vi "QUBE2 RW.vi"(0 "QFLEX Cluster In":T1={"Error"={"status"=FALSE, "code"=0, "source"=""}, "CS DO Ref"={"myRIO Reference"={"myRIO Model"=enum."Unknown", "myRIO Hardware Reference"={"Generic FPGA Reference"=refnum, "Allow multiple opens"=FALSE}}, "DIO Channels List"=[]}, "SPI Ref"={"myRIO Reference"={"myRIO Model"=enum."Unknown", "myRIO Hardware Reference"={"Generic FPGA Reference"=refnum, "Allow multiple opens"=FALSE}}, "SPI Channels Enum"=enum."Not Connected", "SPI Configuration"={"Frequency [Hz]"=0.0, "Clock Phase"=enum."Leading", "Clock Polarity"=enum."Low", "Data Direction"=enum."Most significant bit first", "Frame Length"=8}}} {"SPI Ref"."SPI Configuration"."Frame Length" min=1 max=16}, 5 "LED Color":u32(colorbox)=16711680, 9 "Motor Voltage":dbl, 11 "Reset":bool) -> (3 "Hardware Info":u16[](array[numeric]), 4 "QFLEX Cluster Out":T1={"Error"={"status"=FALSE, "code"=0, "source"=""}, "CS DO Ref"={"myRIO Reference"={"myRIO Model"=enum."Unknown", "myRIO Hardware Reference"={"Generic FPGA Reference"=refnum, "Allow multiple opens"=FALSE}}, "DIO Channels List"=[]}, "SPI Ref"={"myRIO Reference"={"myRIO Model"=enum."Unknown", "myRIO Hardware Reference"={"Generic FPGA Reference"=refnum, "Allow multiple opens"=FALSE}}, "SPI Channels Enum"=enum."Not Connected", "SPI Configuration"={"Frequency [Hz]"=0.0, "Clock Phase"=enum."Leading", "Clock Polarity"=enum."Low", "Data Direction"=enum."Most significant bit first", "Frame Length"=8}}} {"SPI Ref"."SPI Configuration"."Frame Length" min=1 max=16}, 6 "Encoder (counts)":i32[](array[numeric]), 8 "Encoders (rads)":dbl[](array[numeric]), 10 "Tachometer (rads/s)":dbl, 12 "Stall Error":bool, 15 "Motor Current (mA)":dbl)   [LabVIEW 2016]
uses:
  QFLEX myRIO.ctl
  <vilib>/myRIO/Instrument Drivers/Onboard IO/DIO/typedefs/DIO Reference.ctl
  <vilib>/myRIO/Common/Instrument Driver Framework/Utilities/typedefs/myRIO Generic Hardware Reference.ctl
  <vilib>/myRIO/Common/Instrument Driver Framework/Utilities/typedefs/Hardware Version Enum.ctl
  <vilib>/myRIO/Common/Instrument Driver Framework/Utilities/typedefs/myRIO v1.0 Reference.ctl
  <vilib>/myRIO/Common/Instrument Driver Framework/Utilities/typedefs/Generic FPGA Reference.ctl
  <vilib>/myRIO/Common/Instrument Driver Framework/myRIO v1.0/DIO/typedefs/DIO Channels List.ctl
  <vilib>/myRIO/Common/Instrument Driver Framework/myRIO v1.0/DIO/typedefs/DIO Channels Enum.ctl
  <vilib>/myRIO/Instrument Drivers/Onboard IO/SPI/typedefs/SPI Reference.ctl
  <vilib>/myRIO/Common/Instrument Driver Framework/myRIO v1.0/SPI/typedefs/SPI Channels Enum.ctl
  <vilib>/myRIO/Instrument Drivers/Onboard IO/SPI/typedefs/SPI Configuration.ctl
  <vilib>/myRIO/Common/Instrument Driver Framework/myRIO v1.0/SPI/typedefs/SPI Clock Phase.ctl
  <vilib>/myRIO/Common/Instrument Driver Framework/myRIO v1.0/SPI/typedefs/SPI Clock Polarity.ctl
  <vilib>/myRIO/Common/Instrument Driver Framework/myRIO v1.0/SPI/typedefs/SPI Data Direction.ctl
  <vilib>/myRIO/Common/Instrument Driver Framework/myRIO v1.0/SPI/typedefs/SPI Frame Length.ctl
  <vilib>/Utility/error.llb/Error Cluster From Error Code.vi
  <vilib>/myRIO/Common/Instrument Driver Framework/myRIO v1.0/DIO/vis/myRIO v1.0 Write DIO.vi
  <vilib>/myRIO/Common/Instrument Driver Framework/myRIO v1.0/SPI/vis/myRIO v1.0 Write Read SPI.vi
  <vilib>/myRIO/Instrument Drivers/Onboard IO/SPI/SPI.lvlib
  <vilib>/myRIO/Instrument Drivers/Onboard IO/DIO/DIO.lvlib
panel:
  out "Stall Detect":bool
  out "Amp Error":bool
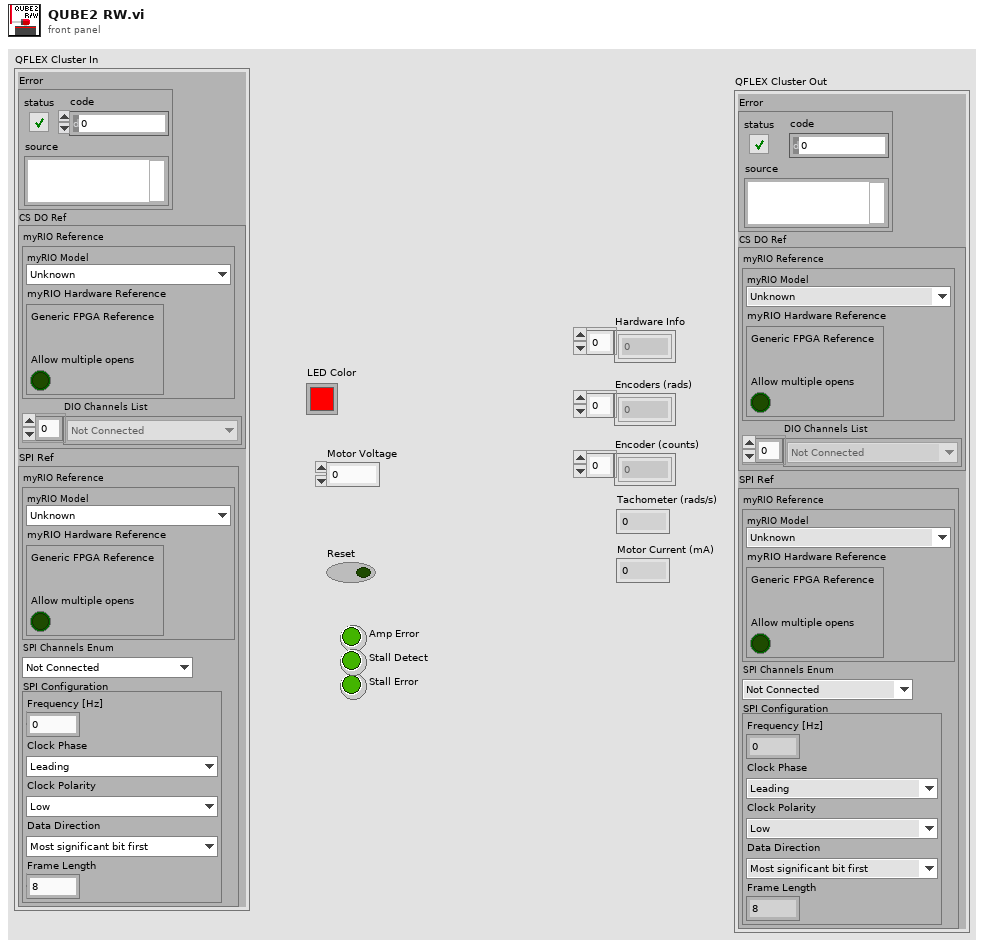
[diagram p1: front panel]
types:
  T1 = typedef "QFLEX myRIO.ctl" = cluster{"Error":errorcluster, "CS DO Ref":T2, "SPI Ref":T9}
  T2 = typedef "DIO.lvlib/DIO Reference.ctl" = cluster{"myRIO Reference":T3, "DIO Channels List":T7}
  T3 = typedef "myRIO Generic Hardware Reference.ctl" = cluster{"myRIO Model":T4, "myRIO Hardware Reference":T5}
  T4 = typedef "Hardware Version Enum.ctl" = enum16{"Unknown", "myRIO-1900", "myRIO-1950", "roboRIO", "NI ELVIS RIO CM"}
  T5 = typedef "myRIO v1.0 Reference.ctl" = cluster{"Generic FPGA Reference":T6, "Allow multiple opens":bool}
  T6 = typedef "Generic FPGA Reference.ctl" = refnum<k20>
  T7 = typedef "DIO Channels List.ctl" = T8[]
  T8 = typedef "DIO Channels Enum.ctl" = enum16{"Not Connected", "C/DIO0", "C/DIO1", "C/DIO2", "C/DIO3", "C/DIO4", "C/DIO5", "C/DIO6", "C/DIO7", "A/DIO0", "A/DIO1", "A/DIO2", "A/DIO3", "A/DIO4", "A/DIO5", "A/DIO6", "A/DIO7", "A/DIO8", "A/DIO9", "A/DIO10", "A/DIO11", "A/DIO12", "A/DIO13", "A/DIO14", "A/DIO15", "B/DIO0", "B/DIO1", "B/DIO2", "B/DIO3", "B/DIO4", "B/DIO5", "B/DIO6", "B/DIO7", "B/DIO8", "B/DIO9", "B/DIO10", "B/DIO11", "B/DIO12", "B/DIO13", "B/DIO14", "B/DIO15", "LED0", "LED1", "LED2", "LED3", "Button0", "DIO/DIO0", "DIO/DIO1", "DIO/DIO2", "DIO/DIO3", "DIO/DIO4", "DIO/DIO5", "DIO/DIO6", "DIO/DIO7", "DIO/DIO8", "DIO/DIO9", "SPI/CS0", "SPI/CS1", "SPI/CS2", "SPI/CS3", "LED RADIO (Green)", "LED RADIO (Red)", "LED COMM (Green)", "LED COMM (Red)", "LED MODE (Green)", "LED MODE (Red)"}
  T9 = typedef "SPI.lvlib/SPI Reference.ctl" = cluster{"myRIO Reference":T3, "SPI Channels Enum":T10, "SPI Configuration":T11}
  T10 = typedef "SPI Channels Enum.ctl" = enum16{"Not Connected", "A/SPI", "B/SPI", "SPI/SPI"}
  T11 = typedef "SPI.lvlib/SPI Configuration.ctl" = cluster{"Frequency [Hz]":dbl, "Clock Phase":T12, "Clock Polarity":T13, "Data Direction":T14, "Frame Length":T15}
  T12 = typedef "SPI Clock Phase.ctl" = enum8{"Leading", "Trailing"}
  T13 = typedef "SPI Clock Polarity.ctl" = enum8{"Low", "High"}
  T14 = typedef "SPI Data Direction.ctl" = enum8{"Most significant bit first", "Least significant bit first"}
  T15 = typedef "SPI Frame Length.ctl" = u8
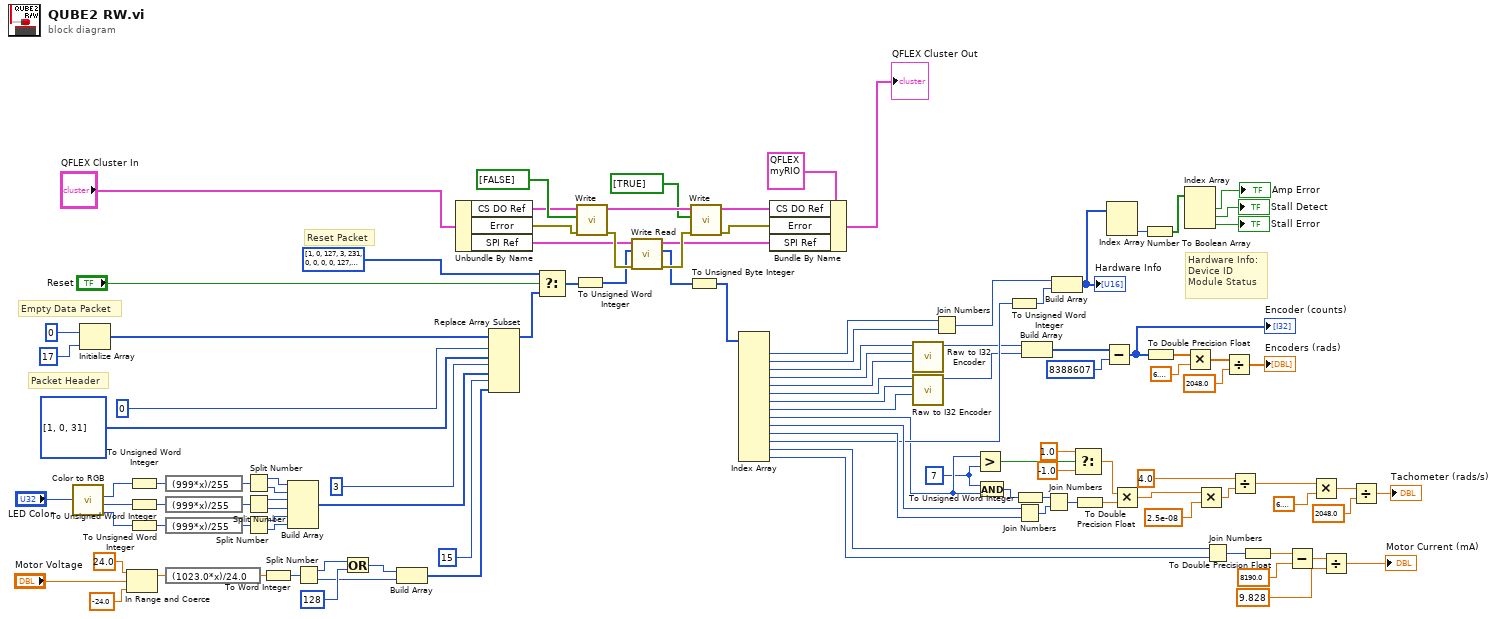
[diagram p0: block diagram]
diagram:
  w46 = u8 7 ("x")
  # "Reset Packet"
  # "Hardware Info:\nDevice ID\nModule Status"
  # "Empty Data Packet"
  # "Packet Header"
  n1 = call <vilib>:"Color to RGB.vi"("Color"="LED Color") -> ("R"=w107:u8, "G"=w100:u8, "B"=w99:u8)  [unwired: 1 out]
  n2 = Initialize Array(u8 0, 17 ("dimension size")) -> (w111:u8[])
  n3 = In Range and Coerce(upper limit=24.0, x="Motor Voltage", lower limit=-24.0) -> (coerced(x)=w36:dbl)  [unwired: 1 out]
  n4 = To Unsigned Word Integer(number=w107) -> (unsigned 16bit integer=w106:u16)
  n5 = To Unsigned Word Integer(number=w100) -> (unsigned 16bit integer=w104:u16)
  n6 = To Unsigned Word Integer(number=w99) -> (unsigned 16bit integer=w102:u16)
  n7 = expression code="(999*x)/255"(w106) -> (w105:u16)
  n8 = expression code="(999*x)/255"(w104) -> (w103:u16)
  n9 = expression code="(999*x)/255"(w102) -> (w101:u16)
  n10 = expression code="(1023.0*x)/24.0"(w36) -> (w89:dbl)
  n11 = Split Number(x=w105) -> (hi(x)=w93:u8, lo(x)=w94:u8)
  n12 = Split Number(x=w103) -> (hi(x)=w95:u8, lo(x)=w96:u8)
  n13 = Split Number(x=w101) -> (hi(x)=w97:u8, lo(x)=w98:u8)
  n14 = To Word Integer(number=w89) -> (16bit integer=w70:i16)
  n15 = Build Array(w93, w94, w95, w96, w97, w98) -> (w91:u8[])
  n16 = Split Number(x=w70) -> (hi(x)=w88:u8, lo(x)=w86:u8)
  n17 = Or(x=w88, y=u8 128) -> (x .or. y?=w85:u8)
  n18 = Build Array(w85, w86) -> (w69:u8[])
  n19 = Unbundle By Name("QFLEX Cluster In") -> ("CS DO Ref"=w23:T2, "Error"=w22:errorcluster, "SPI Ref"=w21:T9)
  n20 = Replace Array Subset(array=w111, new element #1=u8[] [1, 0, 31], index #1=0 ("dimension size"), new element #2=w91, index #2=3 ("dimension size"), new element #3=w69, index #3=15 ("dimension size")) -> (w77:u8[])
  n21 = Select(t=u8[] [1, 0, 127, 3, 231, 0, 0, 0, 0, 127, 255, 255, 127, 255, 255, 0, 0], s="Reset", f=w77) -> (s? t:f=w28:u8[])
  n22 = To Unsigned Word Integer(number=w28) -> (unsigned 16bit integer=w25:u16[])
  n23 = call <vilib>:"Write.vi"("error in (no error)"=w22, "Values"=bool[] [FALSE], "DIO Ref In"=w23) -> ("error out"=w33:errorcluster, "DIO Ref Out"=w32:T2)  [unwired: 6 in]
  n24 = call <vilib>:"Write Read.vi"("error in (no error)"=w33, "Frames to Write"=w25, "SPI Ref In"=w21) -> ("error out"=w31:errorcluster, "Frames Read"=w27:u16[], "SPI Ref Out"=w17:T9)  [unwired: 6 in]
  n25 = To Unsigned Byte Integer(number=w27) -> (unsigned 8bit integer=w26:u8[])
  n26 = call <vilib>:"Write.vi"("error in (no error)"=w31, "Values"=bool[] [TRUE], "DIO Ref In"=w32) -> ("error out"=w18:errorcluster, "DIO Ref Out"=w19:T2)  [unwired: 6 in]
  n27 = Index Array(array=w26) -> (element #1=w79:u8, element #2=w80:u8, element #3=w9:u8, element #4=w8:u8, element #5=w7:u8, element #6=w5:u8, element #7=w4:u8, element #8=w3:u8, element #9=w47:u8, element #10=w82:u8, element #11=w81:u8, element #12=w66:u8, element #13=w65:u8, element #14=w64:u8)  [unwired: 14 in]
  n28 = Bundle By Name(cluster=T1 {"Error"={"status"=FALSE, "code"=0, "source"=""}, "CS DO Ref"={"myRIO Reference"={"myRIO Model"=enum."Unknown", "myRIO Hardware Reference"={"Generic FPGA Reference"=refnum, "Allow multiple opens"=FALSE}}, "DIO Channels List"=[]}, "SPI Ref"={"myRIO Reference"={"myRIO Model"=enum."Unknown", "myRIO Hardware Reference"={"Generic FPGA Reference"=refnum, "Allow multiple opens"=FALSE}}, "SPI Channels Enum"=enum."Not Connected", "SPI Configuration"={"Frequency [Hz]"=0.0, "Clock Phase"=enum."Leading", "Clock Polarity"=enum."Low", "Data Direction"=enum."Most significant bit first", "Frame Length"=8}}} ("QFLEX Cluster In 2"), "CS DO Ref"=w19, "Error"=w18, "SPI Ref"=w17) -> (→"QFLEX Cluster Out":T1)
  n29 = call "Raw to I32 Encoder.vi"("Low Byte"=w7, "Mid Byte"=w8, "High Byte"=w9) -> ("out"=w6:i32)  [unwired: 8 in]
  n30 = call "Raw to I32 Encoder.vi"("Low Byte"=w3, "Mid Byte"=w4, "High Byte"=w5) -> ("out"=w2:i32)  [unwired: 8 in]
  n31 = Join Numbers(hi=w79, lo=w80) -> ((hi.lo)=w78:u16)
  n32 = Greater?(x=w47, y=w46) -> (0:w45:bool)
  n33 = And(x=w46, y=w47) -> (x .and. y?=w48:u8)
  n34 = To Unsigned Word Integer(number=w66) -> (unsigned 16bit integer=w68:u16)
  n35 = To Unsigned Word Integer(number=w48) -> (unsigned 16bit integer=w83:u16)
  n36 = Join Numbers(hi=w82, lo=w81) -> ((hi.lo)=w84:u16)
  n37 = Build Array(w6, w2) -> (w1:i32[])
  n38 = Join Numbers(hi=w83, lo=w84) -> ((hi.lo)=w44:u32)
  n39 = Build Array(w78, w68) -> (w11:u16[])
  "Hardware Info" <- w11
  n40 = Select(t=1.0, s=w45, f=-1.0) -> (s? t:f=w41:dbl)
  n41 = To Double Precision Float(number=w44) -> (double precision float=w43:dbl)
  n42 = Subtract(x=w1, y=8388607) -> (x-y=w52:i32[])
  "Encoder (counts)" <- w52
  n43 = Index Array ("Index Array 2")(array=w11) -> (element #2=w10:u16)  [unwired: 2 in, 1 out]
  n44 = Multiply(x=w41, y=w43) -> (x*y=w42:dbl)
  n45 = Number To Boolean Array(number=w10) -> (Boolean array=w15:bool[])
  n46 = To Double Precision Float(number=w52) -> (double precision float=w53:dbl[])
  n47 = Index Array ("Index Array 3")(array=w15) -> (element #1=→"Amp Error":bool, element #2=→"Stall Detect":bool, element #3=→"Stall Error":bool)  [unwired: 3 in]
  n48 = Multiply(x=w53, y=6.283185307179586) -> (x*y=w73:dbl[])
  n49 = Multiply(x=w42, y=2.5e-08) -> (x*y=w55:dbl)
  n50 = Join Numbers(hi=w65, lo=w64) -> ((hi.lo)=w63:u16)
  n51 = Divide(x=w73, y=2048.0 ("element")) -> (x/y=→"Encoders (rads)":dbl[])
  n52 = Divide(x=4.0, y=w55) -> (x/y=w56:dbl)
  n53 = To Double Precision Float(number=w63) -> (double precision float=w62:dbl)
  n54 = Subtract(x=w62, y=8190.0) -> (x-y=w60:dbl)
  n55 = Multiply(x=w56, y=6.283185307179586) -> (x*y=w72:dbl)
  n56 = Divide(x=w60, y=9.828) -> (x/y=→"Motor Current (mA)":dbl)
  n57 = Divide(x=w72, y=2048.0 ("element")) -> (x/y=→"Tachometer (rads/s)":dbl)
